vi "Write Digital Display[].vi"(5 "Digital Display[]":refnum<class "Digital.lvclass">[](array[class]), 9 "WaveformChart in":refnum<class "WaveformGraph.lvclass">) -> (3 "WaveformChart out":refnum<class "WaveformGraph.lvclass">)   [LabVIEW 2014, in "Raspberry Pi Compatible Compiler for LabVIEW.lvlib" / "WaveformGraph.lvclass"]
uses:
  WaveformGraph.lvclass
  Digital/Digital.lvclass
  WaveformGraph.lvclass/WaveformGraph.ctl
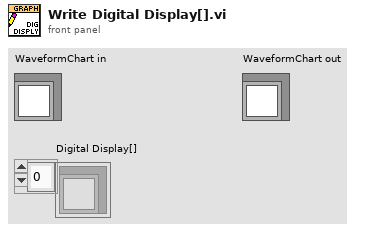
[diagram p1: front panel]
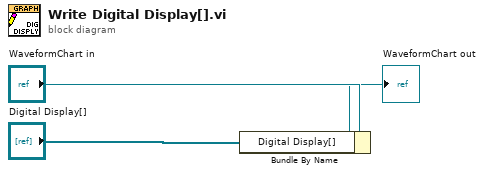
[diagram p0: block diagram]
diagram:
  n1 = Bundle By Name(cluster="WaveformChart in", "Digital Display[]"="Digital Display[]") -> (→"WaveformChart out":refnum<class "WaveformGraph.lvclass">)
